vi "CompositeIterator_Create.vi"(8 "error in (no error)":errorcluster, 11 "reference in":refnum<class "CompositeIterator.lvclass">) -> (0 "error out":errorcluster, 3 "reference out":refnum<class "CompositeIterator.lvclass">)   [LabVIEW 2015, in "CompositeIterator.lvclass"]
uses:
  CompositeIterator.lvclass
  Interface/Iterator.lvclass
  CompositeIterator.lvclass/CompositeIterator.ctl
  ArrayIterator/ArrayIterator.lvclass
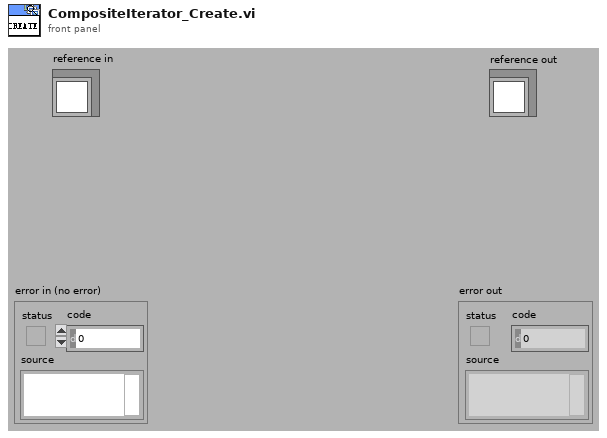
[diagram p1: front panel]
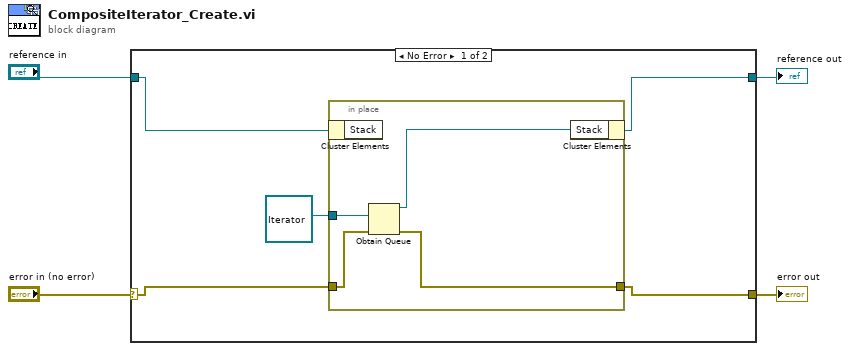
[diagram p0: block diagram]
diagram:
  n1 = case shown="No Error" "error in (no error)" {
    selector: "error in (no error)" -> [w9 w15]
    tunnel: [w8 w15] -> w3
    tunnel: "reference in" -> [w6 w14]
    tunnel: [w5 w14] -> w1
    frame No Error {
      n2 = in-place {
        in-place-border: w9 -> [w12]
        in-place-border: [w13] -> w8
        in-place-border: refnum<class "Iterator.lvclass"> refnum ("Iterator") -> [w11]
        n3 = in-place-cluster #1(w6) -> ()  [unwired: 1 out]
        n4 = Obtain Queue(element data type=w11, error in (no error)=w12) -> (queue out=w10:refnum<queue>, error out=w13:errorcluster)  [unwired: 3 in, 1 out]
        n5 = in-place-cluster #1("Stack"=w10) -> (w5:refnum<class "CompositeIterator.lvclass">)
      }
    }
    frame Error {
    }
  }
  "error out" <- w3
  "reference out" <- w1
